vi "filter7.vi"(6 "initialize":bool, 8 "sampling freq: fs":dbl=1000.0 format="%#_13g", 9 "low cutoff freq: fl":dbl=30.0 format="%0.3f", 11 "Array":dbl[](array[numeric])) -> (3 "appended array":dbl[](array[numeric]))   [LabVIEW 2015]
uses:
  <vilib>/Analysis/3filter.llb/Filter Passband Type.ctl
  <vilib>/ptbypt/NI_PtbyPt.lvlib
  <vilib>/Analysis/NI_AALBase.lvlib
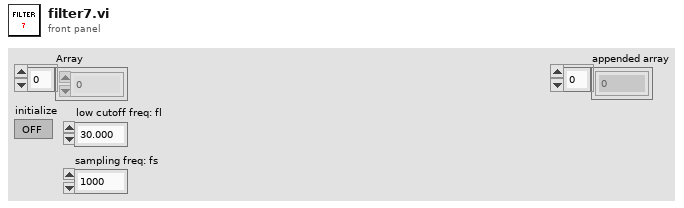
[diagram p1: front panel]
types:
  T1 = typedef "NI_AALBase.lvlib/Filter Passband Type.ctl" = enum32{"Lowpass", "Highpass", "Bandpass", "Bandstop"}
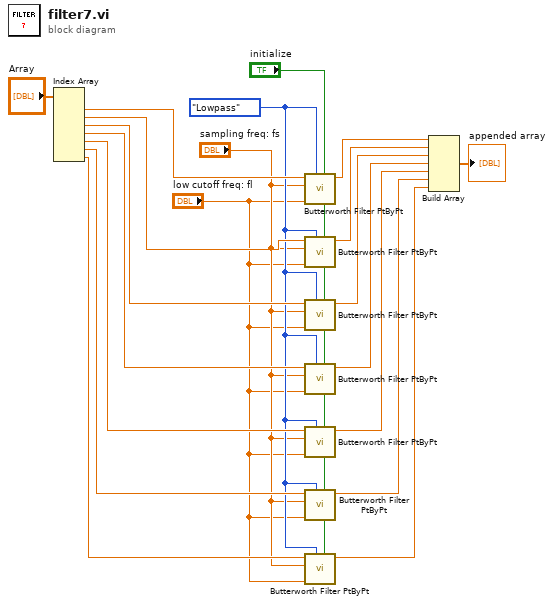
[diagram p0: block diagram]
diagram:
  w6 = Filter_Passband_Type."Lowpass" ("filter type")
  n1 = Index Array(array="Array") -> (element #1=w19:dbl, element #2=w18:dbl, element #3=w17:dbl, element #4=w16:dbl, element #5=w15:dbl, element #6=w14:dbl, element #7=w5:dbl)  [unwired: 7 in]
  n2 = call <vilib>:"Butterworth Filter PtByPt.vi"("initialize"="initialize", "filter type"=w6, "low cutoff freq: fl"="low cutoff freq: fl", "sampling freq: fs"="sampling freq: fs", "x"=w19) -> ("Filtered x"=w13:dbl)  [unwired: 4 in, 1 out]
  n3 = call <vilib>:"Butterworth Filter PtByPt.vi"("initialize"="initialize", "filter type"=w6, "low cutoff freq: fl"="low cutoff freq: fl", "sampling freq: fs"="sampling freq: fs", "x"=w18) -> ("Filtered x"=w12:dbl)  [unwired: 4 in, 1 out]
  n4 = call <vilib>:"Butterworth Filter PtByPt.vi"("initialize"="initialize", "filter type"=w6, "low cutoff freq: fl"="low cutoff freq: fl", "sampling freq: fs"="sampling freq: fs", "x"=w17) -> ("Filtered x"=w11:dbl)  [unwired: 4 in, 1 out]
  n5 = call <vilib>:"Butterworth Filter PtByPt.vi"("initialize"="initialize", "filter type"=w6, "low cutoff freq: fl"="low cutoff freq: fl", "sampling freq: fs"="sampling freq: fs", "x"=w16) -> ("Filtered x"=w10:dbl)  [unwired: 4 in, 1 out]
  n6 = call <vilib>:"Butterworth Filter PtByPt.vi"("initialize"="initialize", "filter type"=w6, "low cutoff freq: fl"="low cutoff freq: fl", "sampling freq: fs"="sampling freq: fs", "x"=w15) -> ("Filtered x"=w9:dbl)  [unwired: 4 in, 1 out]
  n7 = call <vilib>:"Butterworth Filter PtByPt.vi"("initialize"="initialize", "filter type"=w6, "low cutoff freq: fl"="low cutoff freq: fl", "sampling freq: fs"="sampling freq: fs", "x"=w14) -> ("Filtered x"=w8:dbl)  [unwired: 4 in, 1 out]
  n8 = call <vilib>:"Butterworth Filter PtByPt.vi"("initialize"="initialize", "filter type"=w6, "low cutoff freq: fl"="low cutoff freq: fl", "sampling freq: fs"="sampling freq: fs", "x"=w5) -> ("Filtered x"=w7:dbl)  [unwired: 4 in, 1 out]
  n9 = Build Array(w13, w12, w11, w10, w9, w8, w7) -> (→"appended array":dbl[])
